vi "tool_Unicode_Convert ASCII to Unicode.vi"(7 "Source Code Page":T1 items=["System Default"=0, "Thai"=874, "Japanese"=932, "Chinese - Simplified"=936, "Korean"=949, "Chinese - Traditional"=950, "Central Europe"=1250, "Cyrillic"=1251, "Western Europe - Latin"=1252, "Greek"=1253, "Turkish"=1254, "Hebrew"=1255, "Arabic"=1256, "Baltic"=1257, "Vietnamese"=1258, "Unicode UTF-8"=65001], 10 "error in (no error)":errorcluster, 11 "MultiByteStr (ANSI)":string) -> (2 "error out":errorcluster, 3 "WideCharStr (UTF-16LE)":string)   [LabVIEW 2013, in "SET_Unicode Tools.lvlib"]
doc: "tool_Unicode_Convert ANSI to Unicode.vi\n\nConvert Multi-Byte String of a specified code page to UTF-16LE\nunicode string.\n\nThis function calls MultiByteToWideChar from kernel32.dll"
uses:
  SET_Unicode Tools.lvlib
  Code Page List.ctl
  kernel32.dll
panel:
  out "NumWideChars":i32
  # "tool_Unicode_Convert ANSI to Unicode.vi\n\nConvert Multi-Byte String of a specified code page to UTF-16LE\nunicode string.\n\nThis function calls MultiByteToWideChar from kernel32.dll"
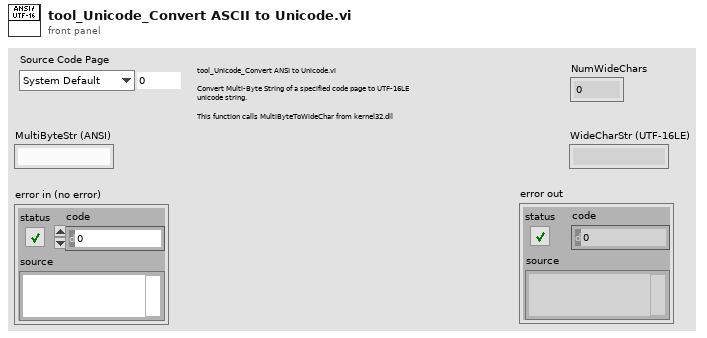
[diagram p1: front panel]
types:
  T1 = typedef "SET_Unicode Tools.lvlib/Code Page List.ctl" = u16
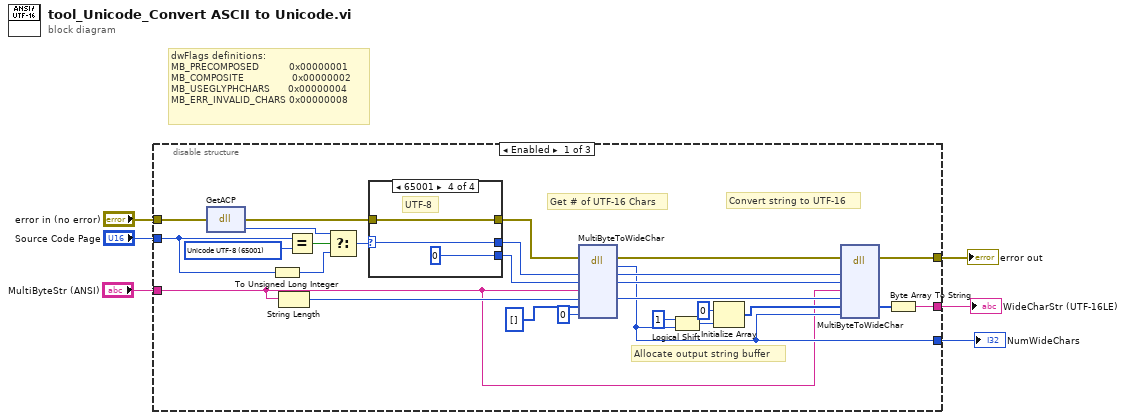
[diagram p0: block diagram]
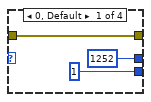
[diagram p2: hidden frame]
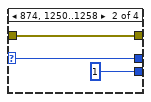
[diagram p3: hidden frame]
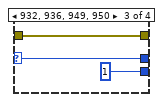
[diagram p4: hidden frame]
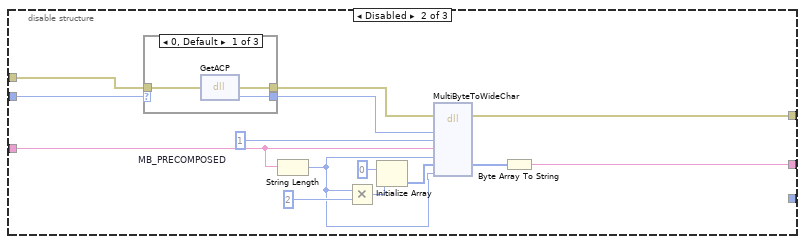
[diagram p5: hidden frame]
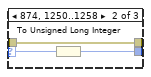
[diagram p6: hidden frame]
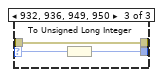
[diagram p7: hidden frame]
diagram:
  # "dwFlags definitions:\nMB_PRECOMPOSED          0x00000001\nMB_COMPOSITE                0x00000002\nMB_USEGLYPHCHARS      0x00000004\nMB_ERR_INVALID_CHARS 0x00000008"
  n1 = disable-structure shown="Enabled" {
    disable-tunnel: "Source Code Page" -> [w24 w53 _]
    disable-tunnel: "MultiByteStr (ANSI)" -> [w7 w52 _]
    disable-tunnel: [w9 w51 _] -> w5
    disable-tunnel: "error in (no error)" -> [w26 w50 _]
    disable-tunnel: [w11 w48 _] -> w3
    disable-tunnel: [w8 _ _] -> w1
    frame Enabled {
      w29 = T1 65001 items=["System Default"=0, "Thai"=874, "Japanese"=932, "Chinese - Simplified"=936, "Korean"=949, "Chinese - Traditional"=950, "Central Europe"=1250, "Cyrillic"=1251, "Western Europe - Latin"=1252, "Greek"=1253, "Turkish"=1254, "Hebrew"=1255, "Arabic"=1256, "Baltic"=1257, "Vietnamese"=1258, "Unicode UTF-8"=65001] ("y")
      # "Allocate output string buffer"
      # "Convert string to UTF-16"
      # "Get # of UTF-16 Chars"
      n2 = dll-call lib="kernel32.dll" fn="GetACP" label="GetACP()"(error in=w26) -> (error out=w22:errorcluster, w25:u32)  [unwired: 2 in, 1 out]
      n3 = To Unsigned Long Integer(number=w24) -> (unsigned 32bit integer=w23:u32)
      n4 = String Length(string=w7) -> (length=w32:i32)
      n5 = Equal?(x=w24, y=w29) -> (x = y?=w27:bool)
      n6 = Select(t=w25, s=w27, f=w23) -> (s? t:f=w28:u32)
      n7 = case shown="65001" w28 {
        selector: w28 -> [_ w38 w41 w44]
        tunnel: [u32 1252 w38 w41 w44] -> w33
        tunnel: w22 -> [w36 w39 w42 w45]
        tunnel: [w36 w39 w42 w45] -> w31
        tunnel: [u32 1 ("MB_PRECOMPOSED") u32 1 ("MB_PRECOMPOSED") u32 1 ("MB_PRECOMPOSED") u32 0 ("NONE")] -> w20
        frame 0, Default {
        }
        frame 874, 1250..1258 {
        }
        frame 932, 936, 949, 950 {
        }
        frame 65001 {
          # "UTF-8"
        }
      }
      n8 = dll-call lib="kernel32.dll" fn="MultiByteToWideChar"(error in=w31, "codePage"=w33, "dwFlags"=w20, "pMultiByteStr"=w7, "cbMultiByte"=w32, "lpWideCharStr"=u8[] [], "cchWideChar"=0) -> (error out=w18:errorcluster, "return type"=w8:i32, "codePage"=w17:u32, "dwFlags"=w16:u32, "cbMultiByte"=w15:i32)  [unwired: 5 in, 1 out]
      n9 = Logical Shift(y=i16 1, x=w8) -> (x << y=w14:i32)
      n10 = Initialize Array(u8 0, w14) -> (w12:u8[])
      n11 = dll-call lib="kernel32.dll" fn="MultiByteToWideChar"(error in=w18, "codePage"=w17, "dwFlags"=w16, "pMultiByteStr"=w7, "cbMultiByte"=w15, "lpWideCharStr"=w12, "cchWideChar"=w8) -> (error out=w9:errorcluster, "lpWideCharStr"=w10:u8[])  [unwired: 7 in, 2 out]
      n12 = Byte Array To String(unsigned byte array=w10) -> (string=w11:string)
    }
    frame Disabled {
      w59 = u32 1  # MB_PRECOMPOSED
      n13 = case shown="0, Default" w53 {
        selector: w53 -> [_ w66 w69]
        tunnel: [w63 w65 w68] -> w54
        tunnel: w50 -> [w62 w64 w67]
        tunnel: [w61 w64 w67] -> w49
        frame 0, Default {
          n14 = dll-call lib="kernel32.dll" fn="GetACP" label="GetACP()"(error in=w62) -> (error out=w61:errorcluster, w63:u32)  [unwired: 2 in, 1 out]
        }
        frame 874, 1250..1258 {
          n15 = To Unsigned Long Integer(number=w66) -> (unsigned 32bit integer=w65:u32)
        }
        frame 932, 936, 949, 950 {
          n16 = To Unsigned Long Integer(number=w69) -> (unsigned 32bit integer=w68:u32)
        }
      }
      n17 = String Length(string=w52) -> (length=w46:i32)
      n18 = Multiply(x=w46, y=2) -> (x*y=w55:i32)
      n19 = Initialize Array(u8 0, w55) -> (w57:u8[])
      n20 = dll-call lib="kernel32.dll" fn="MultiByteToWideChar"(error in=w49, "codePage"=w54, "dwFlags"=w59, "pMultiByteStr"=w52, "cbMultiByte"=w46, "lpWideCharStr"=w57, "cchWideChar"=w46) -> (error out=w51:errorcluster, "return type"=w47:i32, "lpWideCharStr"=w56:u8[])  [unwired: 7 in, 1 out]
      n21 = Byte Array To String(unsigned byte array=w56) -> (string=w48:string)
    }
    frame Disabled {
    }
  }
  "error out" <- w5
  "WideCharStr (UTF-16LE)" <- w3
  "NumWideChars" <- w1
